vi "Apex Valve Compile Data (SubVI).vi"(0 "Waveform Array Input":T2(array[cluster]), 3 "Test Details":T1, 5 "PASS/FAIL":string) -> (17 "XY Graph":cluster{u32[], dbl[]}(graph), 19 "2D Data Array":string[][](array[string]))   [LabVIEW 2009]
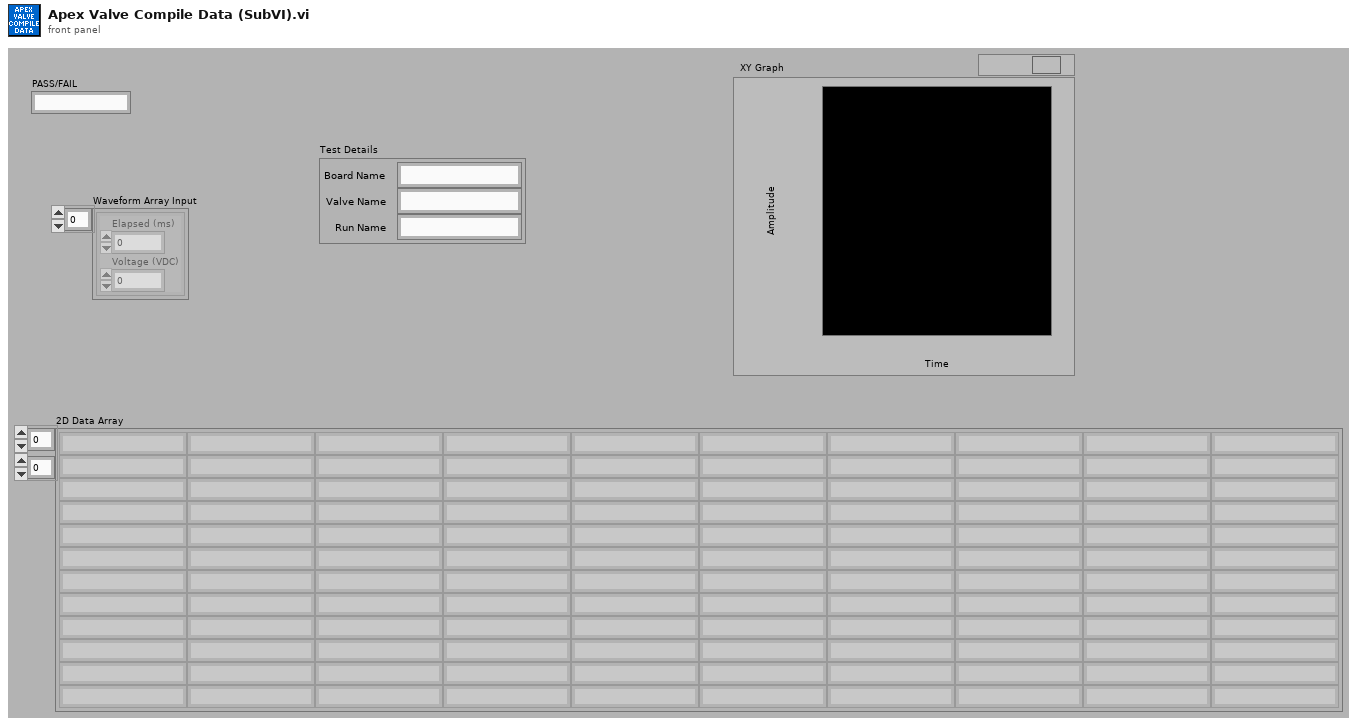
[diagram p1: front panel]
types:
  T1 = cluster{"Board Name":string, "Valve Name":string, "Run Name":string}
  T2 = cluster{"Elapsed (ms)":u32, "Voltage (VDC)":dbl}[]
  T3 = cluster{"TimeStamp":string, "Elapsed (ms)":string, "Voltage (VDC)":string, "Board Name":string, "Valve Name":string, "Run Name":string, "PASS/FAIL":string}
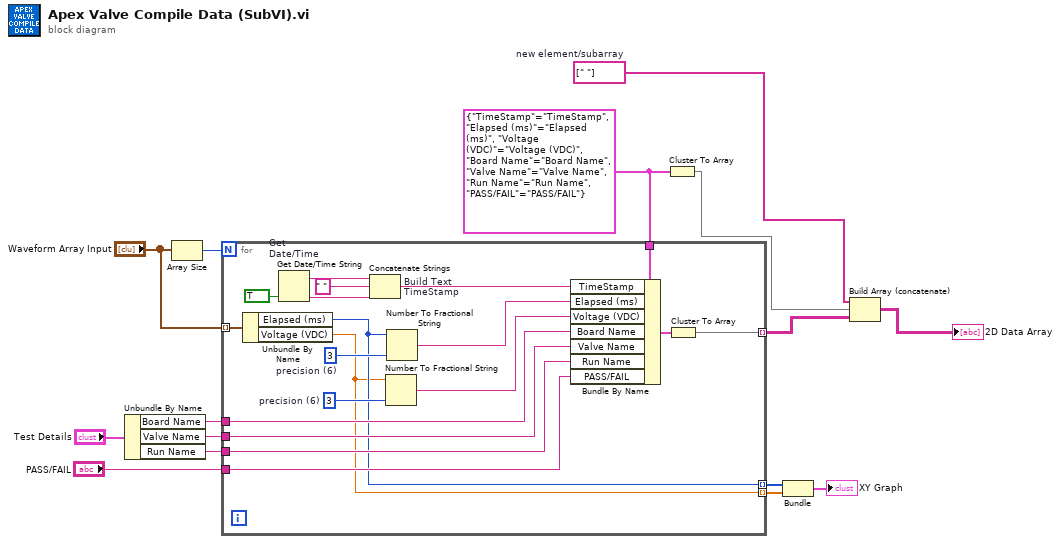
[diagram p0: block diagram]
diagram:
  w4 = string[] [" "]  # new element/subarray
  w5 = T3 {"TimeStamp"="TimeStamp", "Elapsed (ms)"="Elapsed (ms)", "Voltage (VDC)"="Voltage (VDC)", "Board Name"="Board Name", "Valve Name"="Valve Name", "Run Name"="Run Name", "PASS/FAIL"="PASS/FAIL"}
  n1 = Unbundle By Name("Test Details") -> ("Board Name"=w11:string, "Valve Name"=w10:string, "Run Name"=w9:string)
  n2 = Array Size(array="Waveform Array Input") -> (size(s)=w14:i32)
  n3 = for {
    N: w14 -> [_]
    tunnel: "Waveform Array Input" -> [w34] mode=indexing
    tunnel: w5 -> [w33]
    tunnel: w11 -> [w28]
    tunnel: w10 -> [w27]
    tunnel: w9 -> [w26]
    tunnel: [w24] -> w2 mode=indexing
    tunnel: "PASS/FAIL" -> [w23]
    tunnel: [w22] -> w8 mode=indexing
    tunnel: [w21] -> w7 mode=indexing
    w29 = i16 3  # precision (6)
    w31 = i16 3  # precision (6)
    n4 = Unbundle By Name(w34) -> ("Elapsed (ms)"=w22:u32, "Voltage (VDC)"=w21:dbl)
    n5 = Get Date/Time String "Get \nDate/Time"(want seconds? (F)=TRUE) -> (date string=w20:string, time string=w17:string)  [unwired: 2 out]
    n6 = Concatenate Strings "Build Text\nTimeStamp"(w20, " " ("string"), w17) -> (w16:string)
    n7 = Number To Fractional String(number=w21, precision (6)=w29) -> (F-format string=w30:string)  [unwired: 2 in]
    n8 = Number To Fractional String(number=w22, precision (6)=w31) -> (F-format string=w32:string)  [unwired: 2 in]
    n9 = Bundle By Name(cluster=w33, "TimeStamp"=w16, "Elapsed (ms)"=w32, "Voltage (VDC)"=w30, "Board Name"=w28, "Valve Name"=w27, "Run Name"=w26, "PASS/FAIL"=w23) -> (w25:T3)
    n10 = Cluster To Array(cluster=w25) -> (array=w24:string[])
  }
  n11 = Cluster To Array(cluster=w5) -> (array=w3:string[])
  n12 = Bundle(w8, w7) -> (→"XY Graph":cluster{u32[], dbl[]})  [unwired: 1 in]
  n13 = Build Array (concatenate)(w4, w3, w2) -> (→"2D Data Array":string[][])
